vi "Close Serial Port.vi"(8 "error in (no error)":errorcluster, 10 "Connection ID":i32, 11 "Gantry in":refnum<class "Gantry.lvclass">) -> (0 "error out":errorcluster, 3 "Gantry out":refnum<class "Gantry.lvclass">)   [LabVIEW 2023, in "Gantry.lvclass"]
uses:
  Gantry.lvclass
  Gantry.lvclass/Gantry.ctl
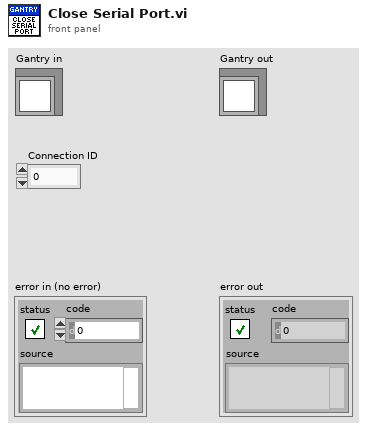
[diagram p1: front panel]
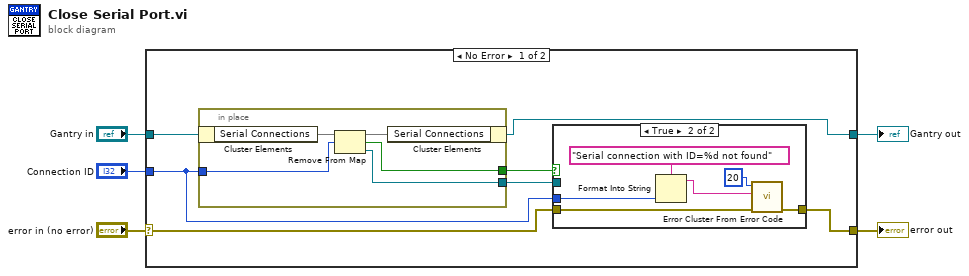
[diagram p0: block diagram]
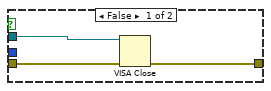
[diagram p2: hidden frame]
diagram:
  n1 = case shown="No Error" "error in (no error)" {
    selector: "error in (no error)" -> [w9 w28]
    tunnel: [w7 w28] -> w4
    tunnel: [w6 w27] -> w2
    tunnel: "Gantry in" -> [w12 w27]
    tunnel: "Connection ID" -> [w8 _]
    frame No Error {
      n2 = in-place {
        in-place-border: w8 -> [w24]
        in-place-border: [w23] -> w10
        in-place-border: [w22] -> w11
        n3 = in-place-cluster #1(w12) -> ("Serial Connections"=w26:map{i32, refnum<visa-resource-name>})
        n4 = Remove From Map(10:w24, 11:w26) -> (1:w23:refnum<visa-resource-name>, 2:w22:bool, 3:w25:map{i32, refnum<visa-resource-name>})
        n5 = in-place-cluster #1("Serial Connections"=w25) -> (w6:refnum<class "Gantry.lvclass">)
      }
      n6 = case shown="True" w11 {
        tunnel: w10 -> [w15 _]
        tunnel: w9 -> [w14 w21]
        tunnel: w8 -> [_ w18]
        tunnel: [w13 w16] -> w7
        frame False {
          n7 = VISA Close(VISA resource name=w15, error in (no error)=w14) -> (error out=w13:errorcluster)
        }
        frame True {
          n8 = Format Into String(format string="Serial connection with ID=%d not found", w18) -> (resulting string=w17:string)  [unwired: 2 in, 1 out]
          n9 = call <vilib>:"Error Cluster From Error Code.vi"("error in (no error)"=w21, "error message (\"\")"=w17, "error code (0)"=20) -> ("error out"=w16:errorcluster)  [unwired: 6 in]
        }
      }
    }
    frame Error {
    }
  }
  "error out" <- w4
  "Gantry out" <- w2
